vi "Init from Config.vi"(7 "Resource":refnum<class "DeployResource.lvclass">, 8 "error in (no error)":errorcluster, 9 "Version":string, 10 "Alias":string, 11 "Device Key":T1) -> (0 "error out":errorcluster, 3 "Device out":refnum<class "Device.lvclass">)   [LabVIEW 2020, in "PicoG-App.lvlib" / "Device.lvclass"]
uses:
  Device.lvclass
  Device Key.ctl
  Builds/picoG/ppl/PicoG-Core.lvlibp/PicoG-Processor/PicoG-Core/DeployResource/DeployResource.lvclass
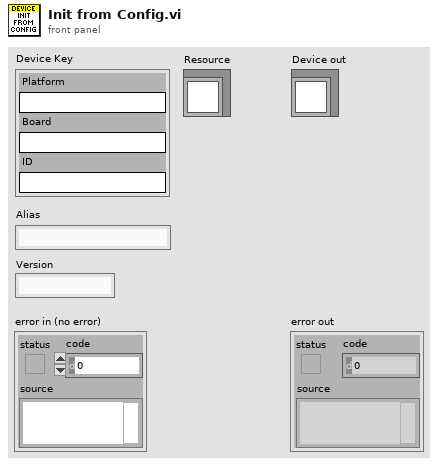
[diagram p1: front panel]
types:
  T1 = typedef "PicoG-App.lvlib/Device.lvclass/Device Key.ctl" = cluster{"Platform":string, "Board":string, "ID":string}
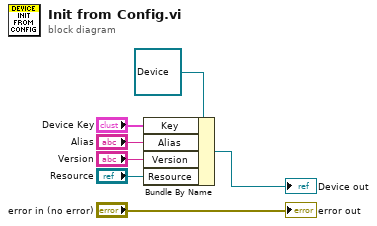
[diagram p0: block diagram]
diagram:
  n1 = Bundle By Name(cluster=refnum<class "Device.lvclass"> refnum ("Device in"), "Key"="Device Key", "Alias"="Alias", "Version"="Version", "Resource"="Resource") -> (→"Device out":refnum<class "Device.lvclass">)
  "error out" <- "error in (no error)"
